vi "LSMcontroller_v65_updatedsealtest.vi"() -> ()   [LabVIEW 2015] (continued)
                                }
                                }
                                }
                                }
                              }
                              frame Enabled {
                              }
                            }
                            n1699 = local write "64bit disabled"(TRUE ("64bit disabled")) -> ()
                          }
                          frame #2 {
                            n1700 = local read "save\ndata"() -> (w4519:bool)
                            n1701 = case shown="True" w4519 {
                              tunnel: w4520 -> [_ w4524]
                              frame False {
                              }
                              frame True {
                                n1702 = local read "filename prefix"() -> (w4522:string)
                                n1703 = local read "data dir"() -> (w4523:path)
                                n1704 = call "preparebinaryfiles.vi"("filename prefix"=w4522, "data dir"=w4523, "timestamp"=w4524) -> ("full-filename"=w4521:string)  [unwired: 1 in]
                                n1705 = local write "full-filename"(w4521) -> ()
                              }
                            }
                            n1706 = call "preptempbuffers_tt.vi"() -> ()  [unwired: 12 in]
                          }
                          frame #3 {
                            n1707 = local read "wavdet"() -> (w4525:bool)
                            n1708 = case shown="False" w4525 {
                              frame False {
                                n1709 = disable-structure shown="Disabled" {
                                frame Disabled {
                                n1710 = call "2pparameters.vi"("command"="get") -> ("params out"=w4527:T10)  [unwired: 1 in]
                                n1711 = Unbundle By Name(w4527) -> ("autoshutter"=w4528:bool)
                                n1712 = case shown="True" w4528 {
                                frame False {
                                }
                                frame True {
                                n1713 = call "shuttercontrol.vi"("command"="open") -> ()  [unwired: 1 in, 1 out]
                                }
                                }
                                }
                                frame Enabled {
                                }
                                }
                              }
                              frame True {
                              }
                            }
                          }
                          frame #4 {
                            n1714 = flat-sequence {
                              frame #0 {
                                # "Disabled for conversion to 64 bit"
                                n1715 = disable-structure shown="Disabled" {
                                frame Disabled {
                                n1716 = local read "Measurement"() -> (w4531:T4)
                                n1717 = case shown="\"Lifetime (contour)\"" w4531 {
                                frame "X-Y-t movie", Default {
                                }
                                frame "Lifetime (contour)" {
                                n1718 = call "runLT_img.vi"() -> ()  [unwired: 1 in]
                                }
                                }
                                }
                                frame Enabled {
                                }
                                }
                                n1719 = local write "64bit disabled"(TRUE ("64bit disabled")) -> ()
                              }
                              frame #1 {
                                n1720 = call "runAI_img.vi"() -> ()  [unwired: 12 in]
                                n1721 = call "runCI.vi"() -> ()  [unwired: 12 in]
                                n1722 = call "runDO_img.vi"() -> ()  [unwired: 12 in]
                              }
                              frame #2 {
                                n1723 = call "runAO_img.vi"() -> ()  [unwired: 12 in]
                              }
                            }
                          }
                          frame #5 {
                            # "Disabled for conversion to 64 bit"
                            n1724 = disable-structure shown="Disabled" {
                              disable-tunnel: w4533 -> [w4534 _]
                              frame Disabled {
                                w4537 = u16 0 items=["Stream to disk", "Post process", "real time process"] ("Ring")
                                n1725 = local read "T3R Data processing"() -> (w4536:u16)
                                n1726 = Equal?(x=w4536, y=w4537) -> (x = y?=w4535:bool)
                                n1727 = local read "save\ndata"() -> (w4539:bool)
                                n1728 = local read "Measurement"() -> (w4540:T4)
                                n1729 = And(x=w4539, y=w4535) -> (x .and. y?=w4538:bool)
                                n1730 = case shown="\"Lifetime (contour)\"" w4540 {
                                tunnel: w4534 -> [_ w4544]
                                tunnel: w4538 -> [_ w4542]
                                frame "X-Y-t movie", Default {
                                }
                                frame "Lifetime (contour)" {
                                n1731 = case shown="True" w4542 {
                                selector: w4542 -> [w4545 w4550]
                                tunnel: w4544 -> [_ w4548]
                                tunnel: [path "" ("appended path") w4551] -> w4543
                                tunnel: [w4545 w4550] -> w4541
                                frame False {
                                }
                                frame True {
                                n1732 = local read "filename prefix"() -> (w4549:string)
                                n1733 = local read "data dir"() -> (w4552:path)
                                n1734 = call "generatedatafilename.vi"("timestamp"=w4548, "filename prefix in"=w4549) -> ("full-filename"=w4547:string)
                                n1735 = Concatenate Strings(w4547, ".lvpt3contour" ("string")) -> (w4554:string)
                                n1736 = Build Path(base path=w4552, name or relative path=w4554) -> (appended path=w4551:path)
                                }
                                }
                                n1737 = call "collectLT_res_v1.vi"("stream?"=w4541, "data file"=w4543) -> ()  [unwired: 2 out]
                                }
                                }
                              }
                              frame Enabled {
                              }
                            }
                            n1738 = while {
                              i -> [w4557]
                              stop <- w4555 stop-if-true
                              n1739 = local read "Stop"() -> (w4565:bool)
                              n1740 = local read "Exit"() -> (w4564:bool)
                              n1741 = Increment(x=w4557) -> (x+1=w4556:i32)
                              n1742 = local write "points recorded"(w4556) -> ()
                              n1743 = Or(x=w4565, y=w4564) -> (x .or. y?=w4563:bool)
                              n1744 = case shown="False" w4563 {
                                frame False {
                                n1745 = stacked-sequence {
                                frame #0 {
                                n1746 = call "collectAI_tt_V2.vi"() -> ()  [unwired: 4 in]
                                n1747 = call "collectCI_tt.vi"() -> ("size(s)"=w4572:i32)  [unwired: 3 in]
                                n1748 = local write "scol"(w4572) -> ()
                                }
                                frame #1 {
                                n1749 = local read "Live"() -> (w4573:bool)
                                n1750 = case shown="True" w4573 {
                                frame False {
                                }
                                frame True {
                                n1751 = local read "graph1list"() -> (w4580:u16)
                                n1752 = local read "graph2list"() -> (w4579:u16)
                                n1753 = To Unsigned Word Integer(number=w4580) -> (unsigned 16bit integer=w4578:u16)
                                n1754 = To Unsigned Word Integer(number=w4579) -> (unsigned 16bit integer=w4577:u16)
                                n1755 = call "dattotrace.vi"("graph2list"=w4577, "Current Average"=sgl 1.0, "graph1list"=w4578) -> ("trace2array out"=w4575:sgl[], "trace1array out"=w4586:sgl[])
                                n1756 = local read "bin"() -> (w4587:dbl)
                                n1757 = script code="data=reshape(datain,[bin length(datain)./bin]);\ndataout=mean(data,1);\ndata2=reshape(datain2,[bin length(datain2)./bin]);\ndataout2=mean(data2,1);"("bin"=w4587, "datain"=w4586, "datain2"=w4575) -> ("dataout"=w4585:dbl[], "dataout2"=w4574:dbl[])  [unwired: 1 in, 1 out]
                                n1758 = Array Size(array=w4574) -> (size(s)=w4588:i32)
                                n1759 = Divide(x=w4588, y=2) -> (x/y=w4590:dbl)
                                n1760 = Round To Nearest(number=w4590) -> (nearest integer value=w4592:dbl)
                                n1761 = Array Size(array=w4585) -> (size(s)=w4597:i32)
                                n1762 = Delete From Array(array=w4574, length=w4592, index=0) -> (deleted portion=w4583:dbl[], array with subset deleted=w4584:dbl[])
                                n1763 = Divide(x=w4597, y=2) -> (x/y=w4595:dbl)
                                n1764 = Round To Nearest(number=w4595) -> (nearest integer value=w4593:dbl)
                                n1765 = Delete From Array(array=w4585, length=w4593, index=0) -> (deleted portion=w4582:dbl[], array with subset deleted=w4581:dbl[])
                                n1766 = local write "graph2"(w4581) -> ()
                                n1767 = local write "graph1"(w4582) -> ()
                                n1768 = local write "graph3"(w4583) -> ()
                                n1769 = local write "graph4"(w4584) -> ()
                                }
                                }
                                }
                                frame #2 {
                                n1770 = local read "save\ndata"() -> (w4598:bool)
                                n1771 = case shown="True" w4598 {
                                frame False {
                                }
                                frame True {
                                n1772 = call "savebinaryfiles.vi"() -> ()  [unwired: 1 in]
                                }
                                }
                                }
                                }
                                }
                                frame True {
                                }
                              }
                              n1773 = local read "continuous"() -> (w4560:bool)
                              n1774 = case shown="False" w4560 {
                                tunnel: w4556 -> [w4570 _]
                                tunnel: [w4569 FALSE] -> w4558
                                frame False {
                                n1775 = call "2pparameters.vi"("command"="get") -> ("params out"=w4567:T10)  [unwired: 1 in]
                                n1776 = Unbundle By Name(w4567) -> ("tt_cycles"=w4566:i32)
                                n1777 = Greater Or Equal?(x=w4570, y=w4566) -> (x >= y?=w4569:bool)
                                }
                                frame True {
                                }
                              }
                              n1778 = local read "Stop"() -> (w4562:bool)
                              n1779 = local read "Exit"() -> (w4561:bool)
                              n1780 = Or(x=w4562, y=w4561) -> (x .or. y?=w4559:bool)
                              n1781 = Or(x=w4559, y=w4558) -> (x .or. y?=w4555:bool)
                            }
                            n1782 = local write "64bit disabled"(TRUE ("64bit disabled")) -> ()
                          }
                          frame #6 {
                            # "Disabled for conversion to 64 bit"
                            n1783 = local read "Measurement"() -> (w4601:T4)
                            n1784 = disable-structure shown="Disabled" {
                              disable-tunnel: w4601 -> [w4603 _]
                              disable-tunnel: w4600 -> [w4602 _]
                              frame Disabled {
                                n1785 = case shown="\"Lifetime (contour)\"" w4603 {
                                tunnel: w4602 -> [_ w4604]
                                frame "X-Y-t movie", Default {
                                }
                                frame "Lifetime (contour)" {
                                n1786 = stacked-sequence {
                                tunnel: w4604 -> [_ w4605]
                                frame #0 {
                                n1787 = flat-sequence {
                                frame #0 {
                                n1788 = call "stoperaseLT_img.vi"() -> ()  [unwired: 1 in]
                                }
                                }
                                }
                                frame #1 {
                                w4608 = u16 0 items=["Stream to disk", "Post process", "real time process"] ("Ring")
                                n1789 = local read "T3R Data processing"() -> (w4607:u16)
                                n1790 = local read "save\ndata"() -> (w4610:bool)
                                n1791 = Equal?(x=w4607, y=w4608) -> (x = y?=w4606:bool)
                                n1792 = Not(x=w4606) -> (.not. x?=w4611:bool)
                                n1793 = And(x=w4610, y=w4611) -> (x .and. y?=w4609:bool)
                                n1794 = case shown="True" w4609 {
                                tunnel: w4605 -> [_ w4612]
                                frame False {
                                }
                                frame True {
                                n1795 = local read "filename prefix"() -> (w4613:string)
                                n1796 = local read "data dir"() -> (w4629:path)
                                n1797 = call "2pparameters.vi"("command"="get") -> ("params out"=w4624:T10)  [unwired: 1 in]
                                n1798 = call "generatedatafilename.vi"("timestamp"=w4612, "filename prefix in"=w4613) -> ("full-filename"=w4614:string)
                                n1799 = Unbundle By Name(w4624) -> ("srate"=w4622:sgl, "Pel"=w4621:sgl, "measpoints"=w4619:i32)
                                n1800 = Concatenate Strings(w4614, ".lvpt3contour" ("string")) -> (w4627:string)
                                n1801 = Build Path(base path=w4629, name or relative path=w4627) -> (appended path=w4626:path)
                                n1802 = To Unsigned Long Integer(number=w4622) -> (unsigned 32bit integer=w4623:u32)
                                n1803 = To Unsigned Long Integer(number=w4621) -> (unsigned 32bit integer=w4620:u32)
                                n1804 = To Unsigned Long Integer(number=w4619) -> (unsigned 32bit integer=w4618:u32)
                                n1805 = call "PH-temp-raw.vi"("command"="get") -> ("array out"=w4617:u32[])  [unwired: 1 in]
                                n1806 = Build Array (concatenate)(w4623, w4620, w4618, w4617) -> (w4616:u32[])
                                n1807 = Open/Create/Replace File(file path (use dialog)=w4626, operation (0:open)=T8."replace or create") -> (refnum out=w4633:refnum<file>, error out=w4632:errorcluster)  [unwired: 4 in, 1 out]
                                n1808 = Write to Binary File(file (use dialog)=w4633, data=w4616, error in=w4632, 5:FALSE ("prepend array or string size? (T)")) -> (refnum out=w4630:refnum<file>, error out=w4631:errorcluster)  [unwired: 2 in, 1 out]
                                n1809 = Close File(refnum=w4630, error in=w4631) -> ()  [unwired: 2 out]
                                }
                                }
                                }
                                }
                                }
                                }
                              }
                              frame Enabled {
                              }
                            }
                            n1810 = local write "64bit disabled"(TRUE ("64bit disabled")) -> ()
                          }
                          frame #7 {
                            n1811 = call "reset AO_DO_v3.vi"() -> ()  [unwired: 12 in]
                          }
                          frame #8 {
                            n1812 = stacked-sequence {
                              tunnel: w4649 -> [w4652 _ _ _ _ _]
                              tunnel: w4646 -> [w4651 _ _ _ _ _]
                              tunnel: w4647 -> [w4650 _ _ _ _ _]
                              tunnel: w4648 -> [_ w4701 _ _ _ _]
                              tunnel: w4644 -> [_ w4700 w4755 w4852 _ _]
                              tunnel: w4645 -> [_ w4699 w4754 w4851 _ _]
                              tunnel: w4643 -> [_ _ _ w4850 _ _]
                              tunnel: w4642 -> [_ _ _ w4849 _ _]
                              tunnel: w4641 -> [_ _ w4752 _ _ _]
                              tunnel: w4640 -> [_ _ w4751 _ _ _]
                              tunnel: w4639 -> [_ _ w4749 _ _ _]
                              tunnel: w4638 -> [_ _ w4748 _ _ _]
                              tunnel: w4637 -> [_ _ _ w4847 _ _]
                              tunnel: w4636 -> [_ _ _ w4846 _ _]
                              frame #0 {
                                n1813 = case shown="False" w4652 {
                                tunnel: w4651 -> [_ w4674]
                                tunnel: w4650 -> [_ w4673]
                                frame True {
                                n1814 = stacked-sequence {
                                seq-local: [w4653 _ _] -> [_ w4665 w4670]
                                frame #0 {
                                n1815 = call "configuration.vi"("command"="get") -> ("config out"=w4659:T11)  [unwired: 2 in, 1 out]
                                n1816 = Unbundle By Name(w4659) -> ("Voltage to Xgalvo"=w4656:i32)
                                n1817 = call "2pparameters.vi"("command"="get") -> ("params out"=w4657:T10)  [unwired: 1 in]
                                n1818 = in-place {
                                in-place-border: w4656 -> [w4664]
                                in-place-border: [w4661] -> w4653
                                n1819 = in-place-cluster #31(w4657) -> ("aAO"=w4663:u32[])
                                n1820 = call "remove channel from active arrayv2.vi"("line array in"=w4663, "line to remove"=w4664) -> ("line array out"=w4662:u32[], "index"=w4661:i32)  [unwired: 1 out]
                                n1821 = in-place-cluster #31("aAO"=w4662) -> (w4654:T10)
                                }
                                n1822 = call "2pparameters.vi"("Params in"=w4654, "command"="set") -> ()  [unwired: 1 out]
                                }
                                frame #1 {
                                n1823 = call "waveformparamsv2.vi"("command"="rem AO", "index"=w4665) -> ()  [unwired: 3 in, 3 out]
                                }
                                frame #2 {
                                n1824 = call "waveformsAObuffer.vi"("command"="get") -> ("AO wf out"=w4671:waveform(dbl)[])  [unwired: 1 in]
                                n1825 = Delete From Array(array=w4671, length=1, index=w4670) -> (array with subset deleted=w4667:waveform(dbl)[])  [unwired: 1 out]
                                n1826 = call "waveformsAObuffer.vi"("AO wf in"=w4667, "command"="set") -> ()  [unwired: 1 out]
                                }
                                }
                                }
                                frame False {
                                n1827 = stacked-sequence {
                                seq-local: [w4675 _ _] -> [_ w4683 w4694]
                                tunnel: w4674 -> [_ w4682 _]
                                tunnel: w4673 -> [_ _ w4693]
                                frame #0 {
                                n1828 = call "configuration.vi"("command"="get") -> ("config out"=w4680:T11)  [unwired: 2 in, 1 out]
                                n1829 = Unbundle By Name(w4680) -> ("Voltage to Xgalvo"=w4676:i32)
                                n1830 = call "2pparameters.vi"("command"="get") -> ("params out"=w4679:T10)  [unwired: 1 in]
                                n1831 = Unbundle By Name(w4679) -> ("aAO"=w4677:u32[])
                                n1832 = Search 1D Array(1D array=w4677, element=w4676) -> (index of element=w4675:i32)  [unwired: 1 in]
                                }
                                frame #1 {
                                n1833 = call "waveformparamsv2.vi"("command"="get") -> ("Params out"=w4686:T14)  [unwired: 4 in, 2 out]
                                n1834 = in-place {
                                in-place-border: w4683 -> [w4690]
                                in-place-border: w4682 -> [w4689]
                                n1835 = in-place-cluster #32(w4686) -> ("AO parameters"=w4691:T15)
                                n1836 = in-place {
                                in-place-border: w4689 -> [w4692]
                                n1837 = in-place-array #33(w4691, w4690) -> ()  [unwired: 1 out]
                                n1838 = in-place-array #33(w4692) -> (w4688:T15)  [unwired: 1 out]
                                }
                                n1839 = in-place-cluster #32("AO parameters"=w4688) -> (w4684:T14)
                                }
                                n1840 = call "waveformparamsv2.vi"("command"="set", "Params in"=w4684) -> ()  [unwired: 3 in, 3 out]
                                }
                                frame #2 {
                                n1841 = call "waveformsAObuffer.vi"("command"="get") -> ("AO wf out"=w4697:waveform(dbl)[])  [unwired: 1 in]
                                n1842 = Replace Array Subset(array=w4697, new element=w4693, index=w4694) -> (w4695:waveform(dbl)[])
                                n1843 = call "waveformsAObuffer.vi"("AO wf in"=w4695, "command"="set") -> ()  [unwired: 1 out]
                                }
                                }
                                }
                                }
                              }
                              frame #1 {
                                n1844 = case shown="False" w4701 {
                                tunnel: w4700 -> [_ w4723]
                                tunnel: w4699 -> [_ w4722]
                                frame True {
                                n1845 = stacked-sequence {
                                seq-local: [w4702 _ _] -> [_ w4714 w4719]
                                frame #0 {
                                n1846 = call "configuration.vi"("command"="get") -> ("config out"=w4708:T11)  [unwired: 2 in, 1 out]
                                n1847 = Unbundle By Name(w4708) -> ("Voltage to Ygalvo"=w4705:i32)
                                n1848 = call "2pparameters.vi"("command"="get") -> ("params out"=w4706:T10)  [unwired: 1 in]
                                n1849 = in-place {
                                in-place-border: w4705 -> [w4713]
                                in-place-border: [w4710] -> w4702
                                n1850 = in-place-cluster #34(w4706) -> ("aAO"=w4712:u32[])
                                n1851 = call "remove channel from active arrayv2.vi"("line array in"=w4712, "line to remove"=w4713) -> ("line array out"=w4711:u32[], "index"=w4710:i32)  [unwired: 1 out]
                                n1852 = in-place-cluster #34("aAO"=w4711) -> (w4703:T10)
                                }
                                n1853 = call "2pparameters.vi"("Params in"=w4703, "command"="set") -> ()  [unwired: 1 out]
                                }
                                frame #1 {
                                n1854 = call "waveformparamsv2.vi"("command"="rem AO", "index"=w4714) -> ()  [unwired: 3 in, 3 out]
                                }
                                frame #2 {
                                n1855 = call "waveformsAObuffer.vi"("command"="get") -> ("AO wf out"=w4720:waveform(dbl)[])  [unwired: 1 in]
                                n1856 = Delete From Array(array=w4720, length=1, index=w4719) -> (array with subset deleted=w4716:waveform(dbl)[])  [unwired: 1 out]
                                n1857 = call "waveformsAObuffer.vi"("AO wf in"=w4716, "command"="set") -> ()  [unwired: 1 out]
                                }
                                }
                                }
                                frame False {
                                n1858 = stacked-sequence {
                                seq-local: [w4724 _ _] -> [_ w4732 w4743]
                                tunnel: w4723 -> [_ w4731 _]
                                tunnel: w4722 -> [_ _ w4742]
                                frame #0 {
                                n1859 = call "configuration.vi"("command"="get") -> ("config out"=w4729:T11)  [unwired: 2 in, 1 out]
                                n1860 = Unbundle By Name(w4729) -> ("Voltage to Ygalvo"=w4725:i32)
                                n1861 = call "2pparameters.vi"("command"="get") -> ("params out"=w4728:T10)  [unwired: 1 in]
                                n1862 = Unbundle By Name(w4728) -> ("aAO"=w4726:u32[])
                                n1863 = Search 1D Array(1D array=w4726, element=w4725) -> (index of element=w4724:i32)  [unwired: 1 in]
                                }
                                frame #1 {
                                n1864 = call "waveformparamsv2.vi"("command"="get") -> ("Params out"=w4735:T14)  [unwired: 4 in, 2 out]
                                n1865 = in-place {
                                in-place-border: w4732 -> [w4739]
                                in-place-border: w4731 -> [w4738]
                                n1866 = in-place-cluster #35(w4735) -> ("AO parameters"=w4740:T15)
                                n1867 = in-place {
                                in-place-border: w4738 -> [w4741]
                                n1868 = in-place-array #36(w4740, w4739) -> ()  [unwired: 1 out]
                                n1869 = in-place-array #36(w4741) -> (w4737:T15)  [unwired: 1 out]
                                }
                                n1870 = in-place-cluster #35("AO parameters"=w4737) -> (w4733:T14)
                                }
                                n1871 = call "waveformparamsv2.vi"("command"="set", "Params in"=w4733) -> ()  [unwired: 3 in, 3 out]
                                }
                                frame #2 {
                                n1872 = call "waveformsAObuffer.vi"("command"="get") -> ("AO wf out"=w4746:waveform(dbl)[])  [unwired: 1 in]
                                n1873 = Replace Array Subset(array=w4746, new element=w4742, index=w4743) -> (w4744:waveform(dbl)[])
                                n1874 = call "waveformsAObuffer.vi"("AO wf in"=w4744, "command"="set") -> ()  [unwired: 1 out]
                                }
                                }
                                }
                                }
                              }
                              frame #2 {
                                n1875 = Build Array(w4752, w4751) -> (w4753:bool[])
                                n1876 = Boolean Array To Number(Boolean array=w4753) -> (number=w4750:u32)
                                n1877 = case shown="2" w4750 {
                                tunnel: w4755 -> [_ _ w4798]
                                tunnel: w4754 -> [_ _ w4797]
                                tunnel: w4749 -> [_ w4777 w4796]
                                tunnel: w4748 -> [_ w4776 w4795]
                                frame 1, Default {
                                n1878 = stacked-sequence {
                                seq-local: [w4756 _ _] -> [_ w4768 w4773]
                                frame #0 {
                                n1879 = call "configuration.vi"("command"="get") -> ("config out"=w4762:T11)  [unwired: 2 in, 1 out]
                                n1880 = Unbundle By Name(w4762) -> ("2P shutter"=w4759:i32)
                                n1881 = call "2pparameters.vi"("command"="get") -> ("params out"=w4760:T10)  [unwired: 1 in]
                                n1882 = in-place {
                                in-place-border: w4759 -> [w4767]
                                in-place-border: [w4764] -> w4756
                                n1883 = in-place-cluster #37(w4760) -> ("aDO"=w4766:u32[])
                                n1884 = call "remove channel from active arrayv2.vi"("line array in"=w4766, "line to remove"=w4767) -> ("line array out"=w4765:u32[], "index"=w4764:i32)  [unwired: 1 out]
                                n1885 = in-place-cluster #37("aDO"=w4765) -> (w4757:T10)
                                }
                                n1886 = call "2pparameters.vi"("Params in"=w4757, "command"="set") -> ()  [unwired: 1 out]
                                }
                                frame #1 {
                                n1887 = call "waveformparamsv2.vi"("command"="rem DO", "index"=w4768) -> ()  [unwired: 3 in, 3 out]
                                }
                                frame #2 {
                                n1888 = call "waveformsDObuffer.vi"("command"="get") -> ("DO wf out"=w4774:digitalwaveform[])  [unwired: 1 in]
                                n1889 = Delete From Array(array=w4774, length=1, index=w4773) -> (array with subset deleted=w4770:digitalwaveform[])  [unwired: 1 out]
                                n1890 = call "waveformsDObuffer.vi"("DO wf in"=w4770, "command"="set") -> ()  [unwired: 1 out]
                                }
                                }
                                }
                                frame 2 {
                                n1891 = stacked-sequence {
                                tunnel: w4777 -> [_ w4788 _]
                                tunnel: w4776 -> [_ _ w4790]
                                frame #0 {
                                n1892 = call "configuration.vi"("command"="get") -> ("config out"=w4779:T11)  [unwired: 2 in, 1 out]
                                n1893 = call "2pparameters.vi"("command"="get") -> ("params out"=w4783:T10)  [unwired: 1 in]
                                n1894 = Unbundle By Name(w4779) -> ("2P shutter"=w4778:i32)
                                n1895 = in-place {
                                in-place-border: w4778 -> [w4787]
                                n1896 = in-place-cluster #38(w4783) -> ("aDO"=w4786:u32[])
                                n1897 = call "add channel to active arrayv2.vi"("line array in"=w4786, "line to add"=w4787) -> ("line array out"=w4785:u32[])  [unwired: 2 out]
                                n1898 = in-place-cluster #38("aDO"=w4785) -> (w4781:T10)
                                }
                                n1899 = call "2pparameters.vi"("Params in"=w4781, "command"="set") -> ()  [unwired: 1 out]
                                }
                                frame #1 {
                                n1900 = call "waveformparamsv2.vi"("command"="add DO", "add DO"=w4788) -> ()  [unwired: 3 in, 3 out]
                                }
                                frame #2 {
                                n1901 = call "waveformsDObuffer.vi"("command"="get") -> ("DO wf out"=w4793:digitalwaveform[])  [unwired: 1 in]
                                n1902 = Build Array (concatenate)(w4793, w4790) -> (w4792:digitalwaveform[])
                                n1903 = call "waveformsDObuffer.vi"("DO wf in"=w4792, "command"="set") -> ()  [unwired: 1 out]
                                }
                                }
                                }
                                frame 0 {
                                n1904 = stacked-sequence {
                                seq-local: [w4799 _ _] -> [_ w4807 w4829]
                                tunnel: w4798 -> [_ _ _]
                                tunnel: w4797 -> [_ _ _]
                                tunnel: w4796 -> [_ w4806 _]
                                tunnel: w4795 -> [_ _ w4828]
                                frame #0 {
                                n1905 = call "configuration.vi"("command"="get") -> ("config out"=w4804:T11)  [unwired: 2 in, 1 out]
                                n1906 = call "2pparameters.vi"("command"="get") -> ("params out"=w4803:T10)  [unwired: 1 in]
                                n1907 = Unbundle By Name(w4804) -> ("2P shutter"=w4800:i32)
                                n1908 = Unbundle By Name(w4803) -> ("aDO"=w4801:u32[])
                                n1909 = Search 1D Array(1D array=w4801, element=w4800) -> (index of element=w4799:i32)  [unwired: 1 in]
                                }
                                frame #1 {
                                n1910 = call "2pparameters.vi"("command"="get") -> ("params out"=w4810:T10)  [unwired: 1 in]
                                n1911 = Unbundle By Name(w4810) -> ("wavdet"=w4808:bool, "autoshutter"=w4809:bool)
                                n1912 = case shown="True" w4809 {
                                tunnel: w4807 -> [_ w4814]
                                tunnel: w4808 -> [_ w4813]
                                tunnel: w4806 -> [_ w4812]
                                frame False {
                                }
                                frame True {
                                n1913 = case shown="False" w4813 {
                                tunnel: w4814 -> [w4818 _]
                                tunnel: w4812 -> [w4815 _]
                                frame False {
                                n1914 = Index Array(array=w4815, index=0) -> (element=w4816:T18)
                                n1915 = call "waveformparamsv2.vi"("command"="get") -> ("Params out"=w4821:T14)  [unwired: 4 in, 2 out]
                                n1916 = in-place {
                                in-place-border: w4818 -> [w4825]
                                in-place-border: w4816 -> [w4823]
                                n1917 = in-place-cluster #39(w4821) -> ("DO parameters"=w4826:T17)
                                n1918 = in-place {
                                in-place-border: w4823 -> [w4827]
                                n1919 = in-place-array #40(w4826, w4825) -> ()  [unwired: 1 out]
                                n1920 = in-place-array #40(w4827) -> (w4824:T17)  [unwired: 1 out]
                                }
                                n1921 = in-place-cluster #39("DO parameters"=w4824) -> (w4819:T14)
                                }
                                n1922 = call "waveformparamsv2.vi"("command"="set", "Params in"=w4819) -> ()  [unwired: 3 in, 3 out]
                                }
                                frame True {
                                }
                                }
                                }
                                }
                                }
                                frame #2 {
                                n1923 = call "2pparameters.vi"("command"="get") -> ("params out"=w4832:T10)  [unwired: 1 in]
                                n1924 = Unbundle By Name(w4832) -> ("wavdet"=w4830:bool, "autoshutter"=w4831:bool)
                                n1925 = case shown="True" w4831 {
                                tunnel: w4829 -> [_ w4836]
                                tunnel: w4830 -> [_ w4835]
                                tunnel: w4828 -> [_ w4834]
                                frame False {
                                }
                                frame True {
                                n1926 = case shown="False" w4835 {
                                tunnel: w4836 -> [w4840 _]
                                tunnel: w4834 -> [w4838 _]
                                frame False {
                                n1927 = Index Array(array=w4838, index=0) -> (element=w4837:digitalwaveform)
                                n1928 = call "waveformsDObuffer.vi"("command"="get") -> ("DO wf out"=w4842:digitalwaveform[])  [unwired: 1 in]
                                n1929 = Replace Array Subset(array=w4842, new element=w4837, index=w4840) -> (w4844:digitalwaveform[])
                                n1930 = call "waveformsDObuffer.vi"("DO wf in"=w4844, "command"="set") -> ()  [unwired: 1 out]
                                }
                                frame True {
                                }
                                }
                                }
                                }
                                }
                                }
                                }
                                }
                              }
                              frame #3 {
                                n1931 = Build Array(w4847, w4846) -> (w4848:bool[])
                                n1932 = Boolean Array To Number(Boolean array=w4848) -> (number=w4845:u32)
                                n1933 = case shown="2" w4845 {
                                tunnel: w4852 -> [_ _ w4895]
                                tunnel: w4851 -> [_ _ w4894]
                                tunnel: w4850 -> [_ w4874 w4892]
                                tunnel: w4849 -> [_ w4873 w4893]
                                frame 1, Default {
                                n1934 = stacked-sequence {
                                seq-local: [w4853 _ _] -> [_ w4865 w4870]
                                frame #0 {
                                n1935 = call "configuration.vi"("command"="get") -> ("config out"=w4859:T11)  [unwired: 2 in, 1 out]
                                n1936 = Unbundle By Name(w4859) -> ("LT timestamp"=w4856:u32)
                                n1937 = call "2pparameters.vi"("command"="get") -> ("params out"=w4857:T10)  [unwired: 1 in]
                                n1938 = in-place {
                                in-place-border: w4856 -> [w4864]
                                in-place-border: [w4861] -> w4853
                                n1939 = in-place-cluster #41(w4857) -> ("aDO"=w4863:u32[])
                                n1940 = call "remove channel from active arrayv2.vi"("line array in"=w4863, "line to remove"=w4864) -> ("line array out"=w4862:u32[], "index"=w4861:i32)  [unwired: 1 out]
                                n1941 = in-place-cluster #41("aDO"=w4862) -> (w4854:T10)
                                }
                                n1942 = call "2pparameters.vi"("Params in"=w4854, "command"="set") -> ()  [unwired: 1 out]
                                }
                                frame #1 {
                                n1943 = call "waveformparamsv2.vi"("command"="rem DO", "index"=w4865) -> ()  [unwired: 3 in, 3 out]
                                }
                                frame #2 {
                                n1944 = call "waveformsDObuffer.vi"("command"="get") -> ("DO wf out"=w4871:digitalwaveform[])  [unwired: 1 in]
                                n1945 = Delete From Array(array=w4871, length=1, index=w4870) -> (array with subset deleted=w4867:digitalwaveform[])  [unwired: 1 out]
                                n1946 = call "waveformsDObuffer.vi"("DO wf in"=w4867, "command"="set") -> ()  [unwired: 1 out]
                                }
                                }
                                }
                                frame 2 {
                                n1947 = stacked-sequence {
                                tunnel: w4874 -> [_ _ w4887]
                                tunnel: w4873 -> [_ w4885 _]
                                frame #0 {
                                n1948 = call "configuration.vi"("command"="get") -> ("config out"=w4876:T11)  [unwired: 2 in, 1 out]
                                n1949 = Unbundle By Name(w4876) -> ("LT timestamp"=w4875:u32)
                                n1950 = call "2pparameters.vi"("command"="get") -> ("params out"=w4880:T10)  [unwired: 1 in]
                                n1951 = in-place {
                                in-place-border: w4875 -> [w4884]
                                n1952 = in-place-cluster #42(w4880) -> ("aDO"=w4883:u32[])
                                n1953 = call "add channel to active arrayv2.vi"("line array in"=w4883, "line to add"=w4884) -> ("line array out"=w4882:u32[])  [unwired: 2 out]
                                n1954 = in-place-cluster #42("aDO"=w4882) -> (w4878:T10)
                                }
                                n1955 = call "2pparameters.vi"("Params in"=w4878, "command"="set") -> ()  [unwired: 1 out]
                                }
                                frame #1 {
                                n1956 = call "waveformparamsv2.vi"("command"="add DO", "add DO"=w4885) -> ()  [unwired: 3 in, 3 out]
                                }
                                frame #2 {
                                n1957 = call "waveformsDObuffer.vi"("command"="get") -> ("DO wf out"=w4890:digitalwaveform[])  [unwired: 1 in]
                                n1958 = Build Array (concatenate)(w4890, w4887) -> (w4889:digitalwaveform[])
                                n1959 = call "waveformsDObuffer.vi"("DO wf in"=w4889, "command"="set") -> ()  [unwired: 1 out]
                                }
                                }
                                }
                                frame 0 {
                                n1960 = stacked-sequence {
                                seq-local: [w4896 _ _] -> [_ w4906 w4923]
                                tunnel: w4895 -> [_ _ _]
                                tunnel: w4894 -> [_ _ _]
                                tunnel: w4893 -> [_ w4903 _]
                                tunnel: w4892 -> [_ _ w4922]
                                frame #0 {
                                n1961 = call "configuration.vi"("command"="get") -> ("config out"=w4901:T11)  [unwired: 2 in, 1 out]
                                n1962 = Unbundle By Name(w4901) -> ("LT timestamp"=w4897:u32)
                                n1963 = call "2pparameters.vi"("command"="get") -> ("params out"=w4900:T10)  [unwired: 1 in]
                                n1964 = Unbundle By Name(w4900) -> ("aDO"=w4898:u32[])
                                n1965 = Search 1D Array(1D array=w4898, element=w4897) -> (index of element=w4896:i32)  [unwired: 1 in]
                                }
                                frame #1 {
                                n1966 = local read "Measurement"() -> (w4905:T4)
                                n1967 = To Unsigned Long Integer(number=w4905) -> (unsigned 32bit integer=w4904:u32)
                                n1968 = case shown="5..7" w4904 {
                                tunnel: w4906 -> [_ w4910]
                                tunnel: w4903 -> [_ w4907]
                                frame 0..4, Default {
                                }
                                frame 5..7 {
                                n1969 = Index Array(array=w4907, index=0) -> (element=w4908:T18)
                                n1970 = call "waveformparamsv2.vi"("command"="get") -> ("Params out"=w4913:T14)  [unwired: 4 in, 2 out]
                                n1971 = in-place {
                                in-place-border: w4910 -> [w4917]
                                in-place-border: w4908 -> [w4915]
                                n1972 = in-place-cluster #43(w4913) -> ("DO parameters"=w4918:T17)
                                n1973 = in-place {
                                in-place-border: w4915 -> [w4919]
                                n1974 = in-place-array #44(w4918, w4917) -> ()  [unwired: 1 out]
                                n1975 = in-place-array #44(w4919) -> (w4916:T17)  [unwired: 1 out]
                                }
                                n1976 = in-place-cluster #43("DO parameters"=w4916) -> (w4911:T14)
                                }
                                n1977 = call "waveformparamsv2.vi"("command"="set", "Params in"=w4911) -> ()  [unwired: 3 in, 3 out]
                                }
                                }
                                }
                                frame #2 {
                                n1978 = local read "Measurement"() -> (w4921:T4)
                                n1979 = To Unsigned Long Integer(number=w4921) -> (unsigned 32bit integer=w4920:u32)
                                n1980 = case shown="5..7" w4920 {
                                tunnel: w4923 -> [_ w4927]
                                tunnel: w4922 -> [_ w4925]
                                frame 0..4, Default {
                                }
                                frame 5..7 {
                                n1981 = Index Array(array=w4925, index=0) -> (element=w4924:digitalwaveform)
                                n1982 = call "waveformsDObuffer.vi"("command"="get") -> ("DO wf out"=w4929:digitalwaveform[])  [unwired: 1 in]
                                n1983 = Replace Array Subset(array=w4929, new element=w4924, index=w4927) -> (w4931:digitalwaveform[])
                                n1984 = call "waveformsDObuffer.vi"("DO wf in"=w4931, "command"="set") -> ()  [unwired: 1 out]
                                }
                                }
                                }
                                }
                                }
                                }
                              }
                              frame #4 {
                                n1985 = call "Used AO lines.vi"() -> ("used AO names"=w4934:string[], "used AO lines"=w4932:tag[])  [unwired: 2 in]
                                n1986 = control-ref of="Analog Lines Plot"() -> (w4933:refnum<vi>)
                                n1987 = control-ref of="Digital Lines Plot"() -> (w4935:refnum<vi>)
                                n1988 = call "Used DO lines.vi"() -> ("used DO names"=w4936:string[], "used DO lines"=w4937:tag[])  [unwired: 2 in]
                                n1989 = local write "Analog Used Lines"(w4932) -> ()
                                n1990 = local write "Analog Used Names"(w4934) -> ()
                                n1991 = local write "Digital Used Lines"(w4937) -> ()
                                n1992 = local write "Digital Used Names"(w4936) -> ()
                                n1993 = call "prepDOWaveplot.vi"("DigitalGraph in"=w4935, "used DO names"=w4936) -> ()  [unwired: 1 in]
                                n1994 = call "prepAOWaveplot.vi"("WaveformGraph in"=w4933, "Analog Used Names"=w4934) -> ()  [unwired: 1 in]
                              }
                              frame #5 {
                                n1995 = local read "Meastab"() -> (w4952:enum32{"X-Y Image", "Linescan", "Timetrace"})
                                n1996 = property on="refwf" class="Ring (strict)"() -> ("RingText.Text"=w4949:string)  [unwired: 2 in, 2 out]
                                n1997 = case shown="\"Timetrace\"" w4952 {
                                tunnel: [w4954 w4955] -> w4953
                                frame "X-Y Image", Default {
                                n1998 = local read "Sampling rate"() -> (w4954:dbl)
                                }
                                frame "Timetrace" {
                                n1999 = local read "srateAODOtt"() -> (w4955:dbl)
                                }
                                }
                                n2000 = call "waveformsAObuffer.vi"("command"="get") -> ("AO wf out"=w4940:waveform(dbl)[])  [unwired: 1 in]
                                n2001 = local read "wavdet"() -> (w4950:bool)
                                n2002 = call "waveformsDObuffer.vi"("command"="get") -> ("DO wf out"=w4944:digitalwaveform[])  [unwired: 1 in]
                                n2003 = call "correctwaveformsizetemp.vi"("new sampling frequency (Hz)"=w4953, "start"=FALSE, "reference waveforms to"=w4949, "Analog waveforms in"=w4940, "stop"=TRUE, "Digital waveforms in"=w4944) -> ("analog wf out"=w4946:waveform(dbl)[], "Digital wf out"=w4948:digitalwaveform[], "measpoints"=w4951:i32)
                                n2004 = local write "Analog Lines Plot"(w4946) -> ()
                                n2005 = call "GetNumCamFramesv2.vi"("Digital Waveform Graph"=w4948) -> ("Numeric"=w4947:i32)  [unwired: 10 in]
                                n2006 = local write "Digital Lines Plot"(w4948) -> ()
                                n2007 = call "waveformsDObuffer.vi"("DO wf in"=w4948, "command"="set") -> ()  [unwired: 1 out]
                                n2008 = call "waveformsAObuffer.vi"("AO wf in"=w4946, "command"="set") -> ()  [unwired: 1 out]
                                n2009 = local write "Total Camera Frames"(w4947) -> ()
                                n2010 = case shown="True" w4950 {
                                tunnel: w4951 -> [_ w4956]
                                frame False {
                                }
                                frame True {
                                n2011 = local write "# of frames"(w4956) -> ()
                                }
                                }
                              }
                            }
                            n2012 = call "stoperaseCI.vi"() -> ()  [unwired: 12 in]
                            n2013 = call "stoperaseDO_img.vi"() -> ()  [unwired: 12 in]
                            n2014 = call "stoperaseAO_img.vi"() -> ()  [unwired: 12 in]
                            n2015 = call "stoperaseAI_img.vi"() -> ()  [unwired: 12 in]
                          }
                          frame #9 {
                            w4966 = FALSE ("Value (Signaling)")
                            n2016 = local read "save\ndata"() -> (w4961:bool)
                            n2017 = case shown="True" w4961 {
                              tunnel: w4960 -> [_ w4973]
                              frame False {
                              }
                              frame True {
                                n2018 = call "closebinaryfiles.vi"() -> ()  [unwired: 12 in]
                                n2019 = local read "filename prefix"() -> (w4975:string)
                                n2020 = local read "data dir"() -> (w4974:path)
                                n2021 = call "saveparams.vi"("timestamp"=w4973, "filename prefix in"=w4975, "data dir in"=w4974) -> ()  [unwired: 1 in]
                              }
                            }
                            n2022 = call "2pparameters.vi"("command"="get") -> ("params out"=w4957:T10)  [unwired: 1 in]
                            n2023 = Unbundle By Name(w4957) -> ("auto OD"=w4958:bool)
                            n2024 = case shown="True" w4958 {
                              frame False {
                              }
                              frame True {
                                n2025 = call "configuration.vi"("command"="get") -> ("config out"=w4969:T11)  [unwired: 2 in, 1 out]
                                n2026 = call "2pparameters.vi"("command"="get") -> ("params out"=w4972:T10)  [unwired: 1 in]
                                n2027 = Unbundle By Name(w4969) -> ("contour OD"=w4967:u16)
                                n2028 = Unbundle By Name(w4972) -> ("ODfilt"=w4968:u16)
                                n2029 = call "filterwheelcontrol_nothorlabslib.vi"("Current OD filt"=w4967, "New ODfilt"=w4968) -> ()  [unwired: 1 in]
                              }
                            }
                            n2030 = property on="Start" class="Bool (strict)"("Val(Sgnl)"=w4966) -> ()  [unwired: 2 in, 2 out]
                            n2031 = property on="Start" class="Bool (strict)"("Visible"=TRUE, "DisabledEnum"=T7."Enabled" ("Disabled")) -> ()  [unwired: 2 in, 2 out]
                            n2032 = property on="Stop" class="Bool (strict)"("Val(Sgnl)"=w4966) -> ()  [unwired: 2 in, 2 out]
                            n2033 = property on="Stop" class="Bool (strict)"("Visible"=FALSE, "DisabledEnum"=T7."Disabled" ("Disabled")) -> ()  [unwired: 2 in, 2 out]
                          }
                          frame #10 {
                            w4978 = T21 2 items=["no dialog", "OK message", "continue or stop message", "OK message + warnings", "continue/stop + warnings"] ("type of dialog (OK msg:1)")
                            n2034 = call "displayerrors.vi"() -> ("error IO"=w4979:errorcluster)
                            n2035 = call <vilib>:"General Error Handler.vi"("type of dialog (OK msg:1)"=w4978, "error in (no error)"=w4979) -> ("error out"=w4977:errorcluster)  [unwired: 9 in, 4 out]
                            n2036 = call <vilib>:"Clear Errors.vi"("error in (no error)"=w4977) -> ("error out"=w4976:errorcluster)  [unwired: 5 in, 1 out]
                            n2037 = call "seterrors.vi"("error IO"=w4976) -> ()
                          }
                        }
                      }
                    }
                  }
                  frame "Lifetime (point)" {
                    # "Disabled for conversion to 64 bit"
                    n2038 = disable-structure shown="Disabled" {
                      frame Disabled {
                        n2039 = stacked-sequence {
                          frame #0 {
                            w4990 = 12.5 ("x")
                            # "get from syncrate"
                            n2040 = local read "Bin size"() -> (w4984:T6)
                            n2041 = local read "Vx-ref"() -> (w4996:dbl)
                            n2042 = local read "Vy-ref"() -> (w4997:dbl)
                            n2043 = call "2pparameters.vi"("command"="get") -> ("params out"=w4982:T10)  [unwired: 1 in]
                            n2044 = Scale By Power Of 2(n=w4984, x=1.0 ("Y Scale.Range:Minimum")) -> (x*2^n=w4993:dbl)
                            n2045 = call "setposition.vi"("Vy"=w4997, "Vx"=w4996) -> ()  [unwired: 1 in]
                            n2046 = Unbundle By Name(w4982) -> ("autoshutter"=w4983:bool)
                            n2047 = Multiply(x=3000.0 ("Y Scale.Range:Minimum"), y=w4993) -> (x*y=w4991:dbl)
                            n2048 = Compound Arithmetic op=MULTIPLY(w4990, invert 3200.0 ("X Scale.Offset and Multiplier:Multiplier"), w4993) -> (w4992:dbl)
                            n2049 = case shown="True" w4983 {
                              frame False {
                              }
                              frame True {
                                n2050 = call "shuttercontrol.vi"("command"="open") -> ()  [unwired: 1 in, 1 out]
                              }
                            }
                            n2051 = call "lifetimeparameters.vi"("command"="get") -> ("Params out"=w4988:T19)  [unwired: 1 in]
                            n2052 = property on="Histogram" class="WFGraph (strict)"("XScale.Maximum"=w4990, "XScale.Minimum"=0.0 ("X Scale.Range:Minimum"), "YScale.Maximum"=w4991, "YScale.Minimum"=0.1 ("Y Scale.Range:Minimum"), "XScale.Multiplier"=w4992) -> ()  [unwired: 2 in, 2 out]
                            n2053 = Bundle By Name(cluster=w4988, "Bin size"=w4984) -> (w4989:T19)
                            n2054 = call "lifetimeparameters.vi"("Params in"=w4989, "command"="set") -> ()  [unwired: 1 out]
                            n2055 = property on="Histogram 2" class="WFGraph (strict)"("YScale.Maximum"=w4991, "XScale.Multiplier"=w4992, "XScale.Maximum"=w4990) -> ()  [unwired: 2 in, 2 out]
                            n2056 = call "2pparameters.vi"("command"="get") -> ("params out"=w5004:T10)  [unwired: 1 in]
                            n2057 = Bundle By Name(cluster=w5004, "type"="Lifetime (point)") -> (w5002:T10)
                            n2058 = property on="Stop" class="Bool (strict)"("Visible"=TRUE, "DisabledEnum"=T7."Enabled" ("Disabled")) -> ()  [unwired: 2 in, 2 out]
                            n2059 = property on="Start" class="Bool (strict)"("Visible"=FALSE, "DisabledEnum"=T7."Disabled and Grayed Out" ("Disabled")) -> ()  [unwired: 2 in, 2 out]
                            n2060 = call "2pparameters.vi"("Params in"=w5002, "command"="set") -> ()  [unwired: 1 out]
                          }
                          frame #1 {
                            n2061 = call "setup.vi"() -> ()  [unwired: 1 in]
                          }
                          frame #2 {
                            # "main loop"
                            n2062 = call "lifetimeparameters.vi"("command"="get") -> ("Params out"=w5014:T19)  [unwired: 1 in]
                            n2063 = Unbundle By Name(w5014) -> ("devidx"=w5012:i32)
                            n2064 = for {
                              N: 10000 -> [_]
                              tunnel: [w5015] -> w5010 mode=indexing
                              i -> [w5015]
                            }
                            n2065 = while {
                              tunnel: w5012 -> [w5019]
                              tunnel: w5010 -> [w5016]
                              i -> [w5017]
                              stop <- w5021 stop-if-true
                              n2066 = Increment(x=w5017) -> (x+1=w5018:i32)
                              n2067 = dll-call lib="phlib.dll" fn="_PH_GetCountRate@8" label="PH_GetCountRate"("devidx"=w5019, "channel"=0) -> (w5020:i32)  [unwired: 5 in, 2 out]
                              "SyncRate" <- w5020
                              n2068 = stacked-sequence {
                                seq-local: [_ _ w5028 _ _] -> [_ _ _ w5041 _]
                                seq-local: [_ _ w5027 _ _] -> [_ _ _ w5040 _]
                                seq-local: [_ w5025 _ _ _] -> [_ _ w5029 _ _]
                                tunnel: w5020 -> [_ _ _ w5048 _]
                                tunnel: w5016 -> [_ _ _ w5038 _]
                                frame #0 {
                                n2069 = call "start_binned.vi"() -> ()  [unwired: 1 in]
                                }
                                frame #1 {
                                n2070 = call "get-histogram.vi"() -> ("IntegralCount"=→"Integral count":u32, "Histogram"=w5025:u32[])
                                "Histogram" <- w5025
                                }
                                frame #2 {
                                n2071 = Search 1D Array(1D array=w5029, element=u32 0) -> (index of element=w5027:i32)  [unwired: 1 in]
                                n2072 = Multiply(x=w5027, y=0.99) -> (x*y=w5033:dbl)
                                n2073 = Array Subset(array=w5029, index=0, length=w5033) -> (w5036:u32[])
                                n2074 = Array Max & Min(array=w5036) -> (max index (indices)=w5030:i32)  [unwired: 3 out]
                                n2075 = Split 1D Array(array=w5036, index=w5030) -> (second subarray=w5032:u32[])  [unwired: 1 out]
                                n2076 = Array Max & Min(array=w5032) -> (min index (indices)=w5031:i32)  [unwired: 3 out]
                                n2077 = Split 1D Array(array=w5032, index=w5031) -> (first subarray=w5028:u32[])  [unwired: 1 out]
                                "Histogram 2" <- w5028
                                }
                                frame #3 {
                                n2078 = Array Size(array=w5041) -> (size(s)=w5043:i32)
                                n2079 = Array Subset(array=w5038, index=0, length=w5043) -> (w5042:i32[])
                                n2080 = Compound Arithmetic op=MULTIPLY(1000000000.0 ("value"), invert w5048, invert w5040, w5042) -> (w5039:dbl[])
                                n2081 = call <vilib>:"Exponential Fit.vi"("Y"=w5041, "X"=w5039) -> ("damping"=w5045:dbl)  [unwired: 8 in, 5 out]
                                n2082 = Divide(x=-1.0 ("y"), y=w5045) -> (x/y=→"Lifetime (ns)":dbl)
                                }
                                frame #4 {
                                n2083 = local read "downright"() -> (w5055:bool)
                                n2084 = local read "downleft"() -> (w5057:bool)
                                n2085 = local read "upright"() -> (w5053:bool)
                                n2086 = local read "upleft"() -> (w5051:bool)
                                n2087 = local read "down"() -> (w5056:bool)
                                n2088 = local read "right"() -> (w5054:bool)
                                n2089 = local read "left"() -> (w5058:bool)
                                n2090 = local read "up"() -> (w5052:bool)
                                n2091 = Compound Arithmetic op=OR(w5051, w5052, w5053, w5054, w5055, w5056, w5057, w5058) -> (w5050:bool)
                                n2092 = case shown="True" w5050 {
                                frame False {
                                }
                                frame True {
                                n2093 = stacked-sequence {
                                frame #0 {
                                n2094 = local read "downright"() -> (w5060:bool)
                                n2095 = local read "downleft"() -> (w5062:bool)
                                n2096 = local read "BigSmall"() -> (w5059:bool)
                                n2097 = local read "upright"() -> (w5064:bool)
                                n2098 = local read "upleft"() -> (w5067:bool)
                                n2099 = local read "down"() -> (w5063:bool)
                                n2100 = local read "right"() -> (w5065:bool)
                                n2101 = local read "left"() -> (w5061:bool)
                                n2102 = local read "up"() -> (w5066:bool)
                                n2103 = call "movestageparams.vi"("command"="get") -> ("Params out"=w5070:T20)  [unwired: 1 in]
                                n2104 = Bundle By Name(cluster=w5070, "upleft"=w5067, "up"=w5066, "upright"=w5064, "right"=w5065, "downright"=w5060, "down"=w5063, "downleft"=w5062, "left"=w5061, "Bigsmall"=w5059) -> (w5071:T20)
                                n2105 = call "movestageparams.vi"("Params in"=w5071, "command"="set") -> ()  [unwired: 1 out]
                                }
                                frame #1 {
                                n2106 = call "movestage.vi"() -> ()  [unwired: 12 in]
                                }
                                frame #2 {
                                w5072 = FALSE ("OK Button")
                                w5073 = FALSE ("OK Button")
                                n2107 = property on="down" class="Bool (strict)"("Value"=w5073) -> ()  [unwired: 2 in, 2 out]
                                n2108 = property on="up" class="Bool (strict)"("Value"=w5073) -> ()  [unwired: 2 in, 2 out]
                                n2109 = property on="right" class="Bool (strict)"("Value"=w5073) -> ()  [unwired: 2 in, 2 out]
                                n2110 = property on="left" class="Bool (strict)"("Value"=w5073) -> ()  [unwired: 2 in, 2 out]
